vi "Projection transformation coefficients from rectangle input and output.vi"(2 "output tetragon":dbl[](array[numeric])=[71.87207560031281, 21.936374908669485, 486.335824943954, 28.133507372302752, 477.67000887595856, 267.4482693053184, 72.8343361065647, 261.0941972226868], 3 "input rectangle":i32[](array[numeric])=[72, 25, 483, 264]) -> (0 "proj trans matrix":dbl[][](array[numeric]), 1 "proj trans coeffs":dbl[](array[numeric])=[-3.137289912322292e-06, 9.961897558771055e-05, 1.009185512099453, 0.011290994215426897, -0.9087953773354798, 0.015024064098859008, 1.0289363657943675, -4.819089966670219] format="%.6f")   [LabVIEW 2024]
uses:
  <vilib>/Analysis/Matrix/Datatypes/RealMatrix.ctl
  <vilib>/Analysis/baseanly.llb/Matrix Type of Inverse Matrix.ctl
  <vilib>/Analysis/baseanly.llb/A x Vector.vi
  <vilib>/Analysis/7linalg.llb/Solve Linear Equations (single right hand).vi
  <vilib>/Analysis/baseanly.llb/Solve Linear Equations By Cholesky.vi
  <vilib>/Analysis/baseanly.llb/Real Matrix to Compact Array.vi
  <vilib>/Analysis/baseanly.llb/Real Compact Tri-Matrix Linear Eqs.vi
  <vilib>/Analysis/baseanly.llb/Real Inverse Matrix.vi
  <vilib>/Analysis/7linalg.llb/Solve Linear Eqs (General).vi
  <vilib>/Analysis/7linalg.llb/Solve Linear Eqs (Gen, single right hand).vi
  <vilib>/Analysis/NI_AALBase.lvlib
  <vilib>/Analysis/NI_AALPro.lvlib
  <vilib>/Analysis/Matrix/NI_Matrix.lvlib
panel:
  out "A x Vector 2":dbl[](array[numeric])=[-1.0, 1.0] format="%.2f"
  in  "Array 2":dbl[](array[numeric])=[1.0, 1.0]
  in  "Array":dbl[][](array[numeric])=[[1.0, 2.0], [3.0, 4.0]]
  out "Inverse Matrix":T1=[[-2.0, 1.0], [1.5, -0.5]]
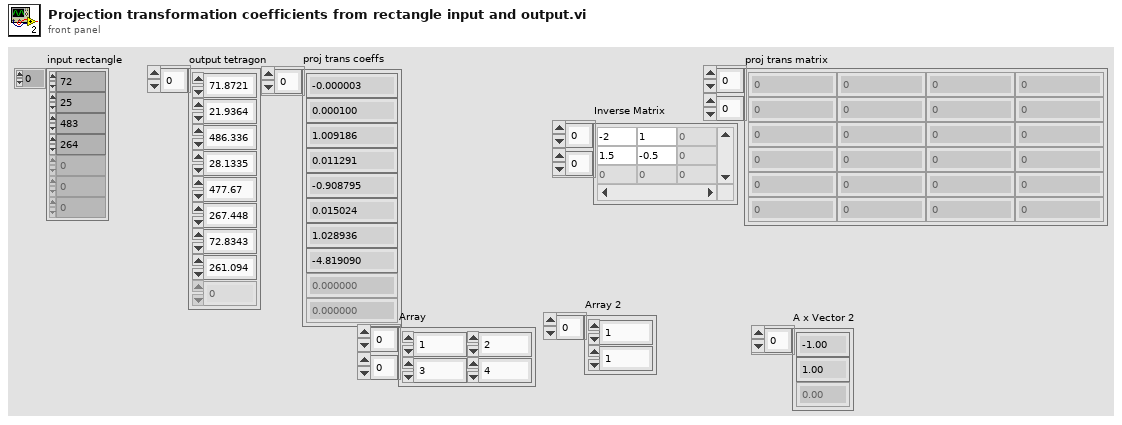
[diagram p1: front panel]
types:
  T1 = typedef "NI_Matrix.lvlib/RealMatrix.ctl" = dbl[][]
  T2 = typedef "NI_AALBase.lvlib/Matrix Type of Inverse Matrix.ctl" = enum32{"General", "Positive Definite", "Lower Triangular", "Upper Triangular"}
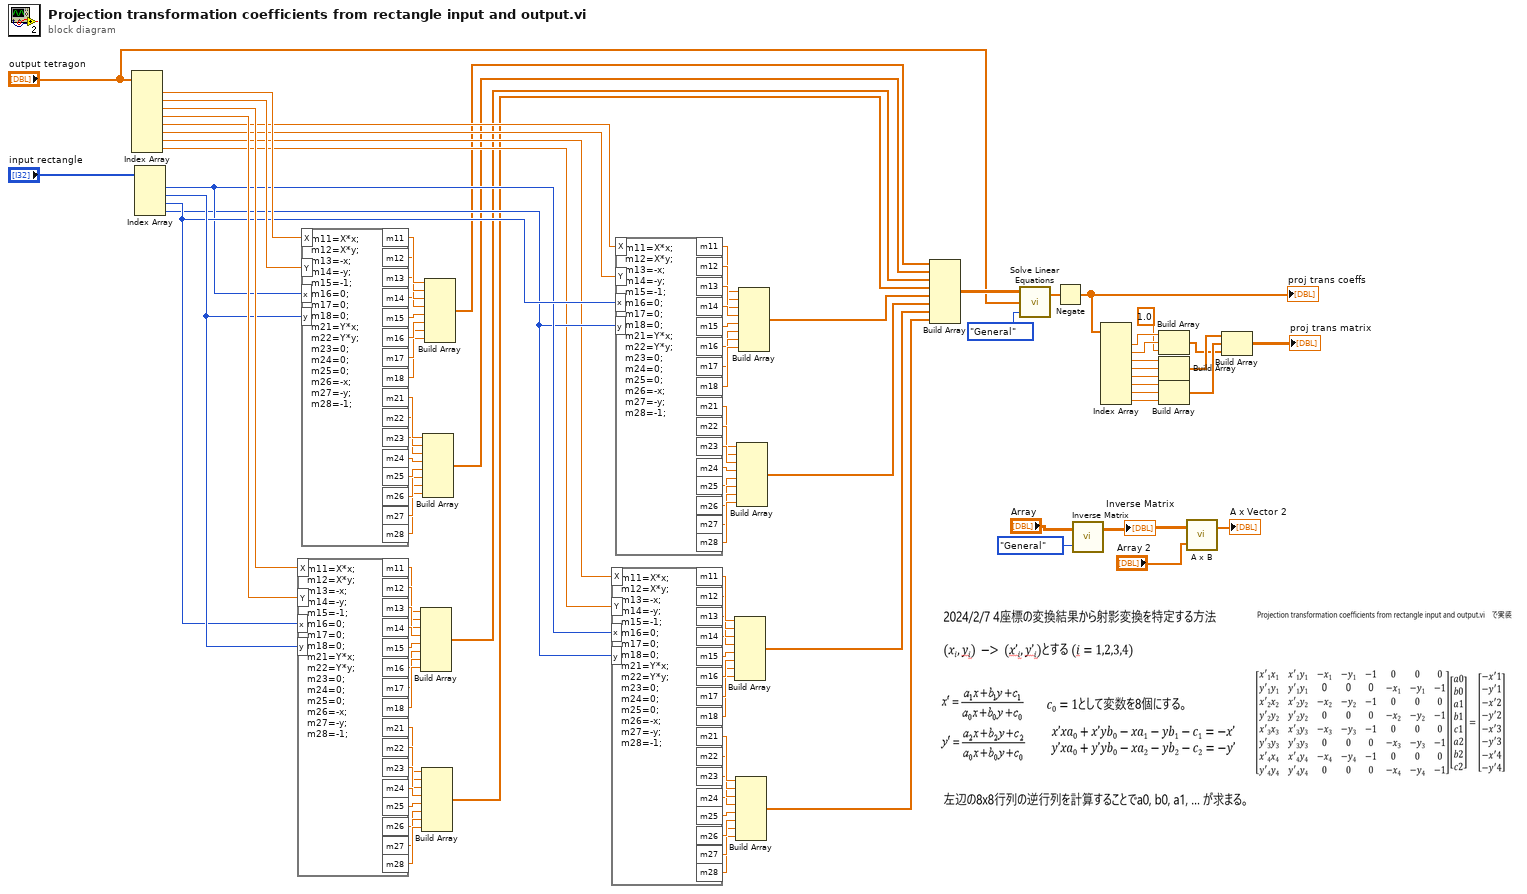
[diagram p0: block diagram]
diagram:
  n1 = Index Array(array="output tetragon") -> (element #1=w91:dbl, element #2=w90:dbl, element #3=w73:dbl, element #4=w72:dbl, element #5=w38:dbl, element #6=w37:dbl, element #7=w33:dbl, element #8=w32:dbl)  [unwired: 8 in]
  n2 = Index Array(array="input rectangle") -> (element #1=w35:i32, element #2=w71:i32, element #3=w36:i32, element #4=w34:i32)  [unwired: 4 in]
  n3 = formula code="m11=X*x;\nm12=X*y;\nm13=-x;\nm14=-y;\nm15=-1;\nm16=0;\nm17=0;\nm18=0;\nm21=Y*x;\nm22=Y*y;\nm23=0;\nm24=0;\nm25=0;\nm26=-x;\nm27=-y;\nm28=-1;"("X"=w73, "Y"=w72, "x"=w36, "y"=w71) -> ("m11"=w74:dbl, "m12"=w75:dbl, "m13"=w76:dbl, "m14"=w77:dbl, "m15"=w78:dbl, "m16"=w79:dbl, "m17"=w80:dbl, "m18"=w81:dbl, "m21"=w82:dbl, "m22"=w83:dbl, "m23"=w84:dbl, "m24"=w85:dbl, "m25"=w86:dbl, "m26"=w87:dbl, "m27"=w88:dbl, "m28"=w89:dbl)
  n4 = formula code="m11=X*x;\nm12=X*y;\nm13=-x;\nm14=-y;\nm15=-1;\nm16=0;\nm17=0;\nm18=0;\nm21=Y*x;\nm22=Y*y;\nm23=0;\nm24=0;\nm25=0;\nm26=-x;\nm27=-y;\nm28=-1;"("X"=w91, "Y"=w90, "x"=w35, "y"=w71) -> ("m11"=w107:dbl, "m12"=w106:dbl, "m13"=w105:dbl, "m14"=w104:dbl, "m15"=w103:dbl, "m16"=w102:dbl, "m17"=w101:dbl, "m18"=w100:dbl, "m21"=w99:dbl, "m22"=w98:dbl, "m23"=w97:dbl, "m24"=w96:dbl, "m25"=w95:dbl, "m26"=w94:dbl, "m27"=w93:dbl, "m28"=w92:dbl)
  n5 = Build Array(w74, w75, w76, w77, w78, w79, w80, w81) -> (w29:dbl[])
  n6 = Build Array(w82, w83, w84, w85, w86, w87, w88, w89) -> (w28:dbl[])
  n7 = Build Array(w99, w98, w97, w96, w95, w94, w93, w92) -> (w30:dbl[])
  n8 = Build Array(w107, w106, w105, w104, w103, w102, w101, w100) -> (w31:dbl[])
  n9 = formula code="m11=X*x;\nm12=X*y;\nm13=-x;\nm14=-y;\nm15=-1;\nm16=0;\nm17=0;\nm18=0;\nm21=Y*x;\nm22=Y*y;\nm23=0;\nm24=0;\nm25=0;\nm26=-x;\nm27=-y;\nm28=-1;"("X"=w33, "Y"=w32, "x"=w35, "y"=w34) -> ("m11"=w70:dbl, "m12"=w69:dbl, "m13"=w68:dbl, "m14"=w67:dbl, "m15"=w66:dbl, "m16"=w65:dbl, "m17"=w64:dbl, "m18"=w63:dbl, "m21"=w62:dbl, "m22"=w61:dbl, "m23"=w60:dbl, "m24"=w59:dbl, "m25"=w58:dbl, "m26"=w57:dbl, "m27"=w56:dbl, "m28"=w55:dbl)
  n10 = formula code="m11=X*x;\nm12=X*y;\nm13=-x;\nm14=-y;\nm15=-1;\nm16=0;\nm17=0;\nm18=0;\nm21=Y*x;\nm22=Y*y;\nm23=0;\nm24=0;\nm25=0;\nm26=-x;\nm27=-y;\nm28=-1;"("X"=w38, "Y"=w37, "x"=w36, "y"=w34) -> ("m11"=w39:dbl, "m12"=w40:dbl, "m13"=w41:dbl, "m14"=w42:dbl, "m15"=w43:dbl, "m16"=w44:dbl, "m17"=w45:dbl, "m18"=w46:dbl, "m21"=w47:dbl, "m22"=w48:dbl, "m23"=w49:dbl, "m24"=w50:dbl, "m25"=w51:dbl, "m26"=w52:dbl, "m27"=w53:dbl, "m28"=w54:dbl)
  n11 = Build Array(w70, w69, w68, w67, w66, w65, w64, w63) -> (w25:dbl[])
  n12 = Build Array(w62, w61, w60, w59, w58, w57, w56, w55) -> (w24:dbl[])
  n13 = Build Array(w47, w48, w49, w50, w51, w52, w53, w54) -> (w26:dbl[])
  n14 = Build Array(w39, w40, w41, w42, w43, w44, w45, w46) -> (w27:dbl[])
  n15 = Build Array(w31, w30, w29, w28, w27, w26, w25, w24) -> (w5:dbl[][])
  n16 = call-poly <vilib>:"Solve Linear Equations.vi"("matrix type"=Matrix_Type_of_Inverse_Matrix."General", "Known Vector"="output tetragon", "Input Matrix"=w5) -> ("Solution Vector"=w2:dbl[])  [unwired: 1 out]
  n17 = Negate(x=w2) -> (-x=w18:dbl[])
  "proj trans coeffs" <- w18
  n18 = call-poly <vilib>:"Inverse Matrix.vi"("matrix type"=Matrix_Type_of_Inverse_Matrix."General", "Input Matrix"="Array") -> ("Inverse Matrix"=w21:T1)  [unwired: 1 out]
  "Inverse Matrix" <- w21
  n19 = Index Array(array=w18) -> (element #1=w17:dbl, element #2=w16:dbl, element #3=w14:dbl, element #4=w13:dbl, element #5=w12:dbl, element #6=w11:dbl, element #7=w10:dbl, element #8=w9:dbl)  [unwired: 8 in]
  n20 = Build Array(w17, w16, 1.0 ("element")) -> (w6:dbl[])
  n21 = Build Array(w14, w13, w12) -> (w8:dbl[])
  n22 = Build Array(w11, w10, w9) -> (w7:dbl[])
  n23 = call-poly <vilib>:"A x B.vi"("Vector"="Array 2", "A"=w21) -> ("A x Vector"=→"A x Vector 2":dbl[])  [unwired: 1 out]
  n24 = Build Array(w8, w7, w6) -> (→"proj trans matrix":dbl[][])
